vi "trace_viewer.vi"() -> ()   [LabVIEW 2012]
uses:
  testing/Trace controls.ctl
  testing/probe_point.ctl
  testing/flag_selector.ctl
  testing/status_flag.ctl
  testing/pose_selector.ctl
  testing/pose_source.ctl
  testing/pose_relative_to.ctl
  ltrace_index.ctl
  bool_condition.ctl
  <vilib>/Platform/TimedLoop/XDataNode/timing_clust.ctl
  <vilib>/Platform/TimedLoop/XDataNode/nitl_modes.ctl
  <vilib>/Platform/TimedLoop/XDataNode/wakeup.ctl
  <vilib>/Platform/TimedLoop/XDataNode/XDataNode.xnode
  <vilib>/Platform/TimedLoop/XDataNode/XDNodeRunTimeDep.lvlib
panel:
  in  "Max len":dbl=120.0
  out "Cursor time":timestamp
  out "Trace display":T1(graph)
  out "Progress":u8(slide) scale=0.0..100.0
  in  "Save trace":bool
  in  "Output path":path
  in  "Show":bool[](array[boolean])=[FALSE, FALSE, TRUE, TRUE, TRUE, FALSE, TRUE, TRUE, TRUE, TRUE, TRUE, FALSE, FALSE, FALSE, FALSE, FALSE, TRUE, TRUE]
  in  "Test":T2[](array[typedef])=[enum."*", enum."1", enum."*", enum."*", enum."*", enum."*", enum."*", enum."*", enum."*", enum."*", enum."*", enum."*", enum."*", enum."*", enum."*", enum."*", enum."*", enum."*"]
  out "Flag names":string[](array[string])
  in  "After":dbl
  in  "Before":dbl
  out "Sequence error":bool
  out "Out of order":i32
  out "Missing":i32
  out "Chunk binary data file":path caption="selected path"
  out "Chunks":cluster{T3[]}[](array[cluster]) {"?"."Timestamp" format="%<%.3X>T"}
  in  "Chunk browser":i32(listbox)
  out "File exists":bool
  in  "Input file":path
  in  "stop":bool
  in  "Reference hold":bool
  in  "Pose selectors":T4[](array[typedef])
  in  "Flag selectors":T7[](array[typedef])=[{"Flag"=enum."Cancellation", "Select"=TRUE}, {"Flag"=enum."Goal filter", "Select"=TRUE}, {"Flag"=enum."Valid position", "Select"=TRUE}, {"Flag"=enum."Velocity limiting", "Select"=TRUE}]
  in  "Decimate":i32=1 min=1 max=999 step=1
  out "2D position":cluster{"X":sgl[], "Y":sgl[]}[](graph)
  in  "Trace controls":T9[](array[typedef])=[{"+ stim"=FALSE, "Relative"=FALSE, "Scale"=enum."1X", "Probe point"=enum."Null pos (tip)", "XYZ selector"={"Boolean"=FALSE, "Boolean 2"=FALSE, "Boolean 3"=TRUE}, "To tip"=TRUE}, {"+ stim"=FALSE, "Relative"=FALSE, "Scale"=enum."1X", "Probe point"=enum."Goal (tip)", "XYZ selector"={"Boolean"=FALSE, "Boolean 2"=FALSE, "Boolean 3"=TRUE}, "To tip"=TRUE}, {"+ stim"=FALSE, "Relative"=FALSE, "Scale"=enum."1X", "Probe point"=enum."Position (tip)", "XYZ selector"={"Boolean"=FALSE, "Boolean 2"=FALSE, "Boolean 3"=TRUE}, "To tip"=TRUE}, {"+ stim"=FALSE, "Relative"=FALSE, "Scale"=enum."1X", "Probe point"=enum."Position (tip)", "XYZ selector"={"Boolean"=FALSE, "Boolean 2"=FALSE, "Boolean 3"=FALSE}, "To tip"=FALSE}]
  # "Trace Display"
  # "Chunk filtering"
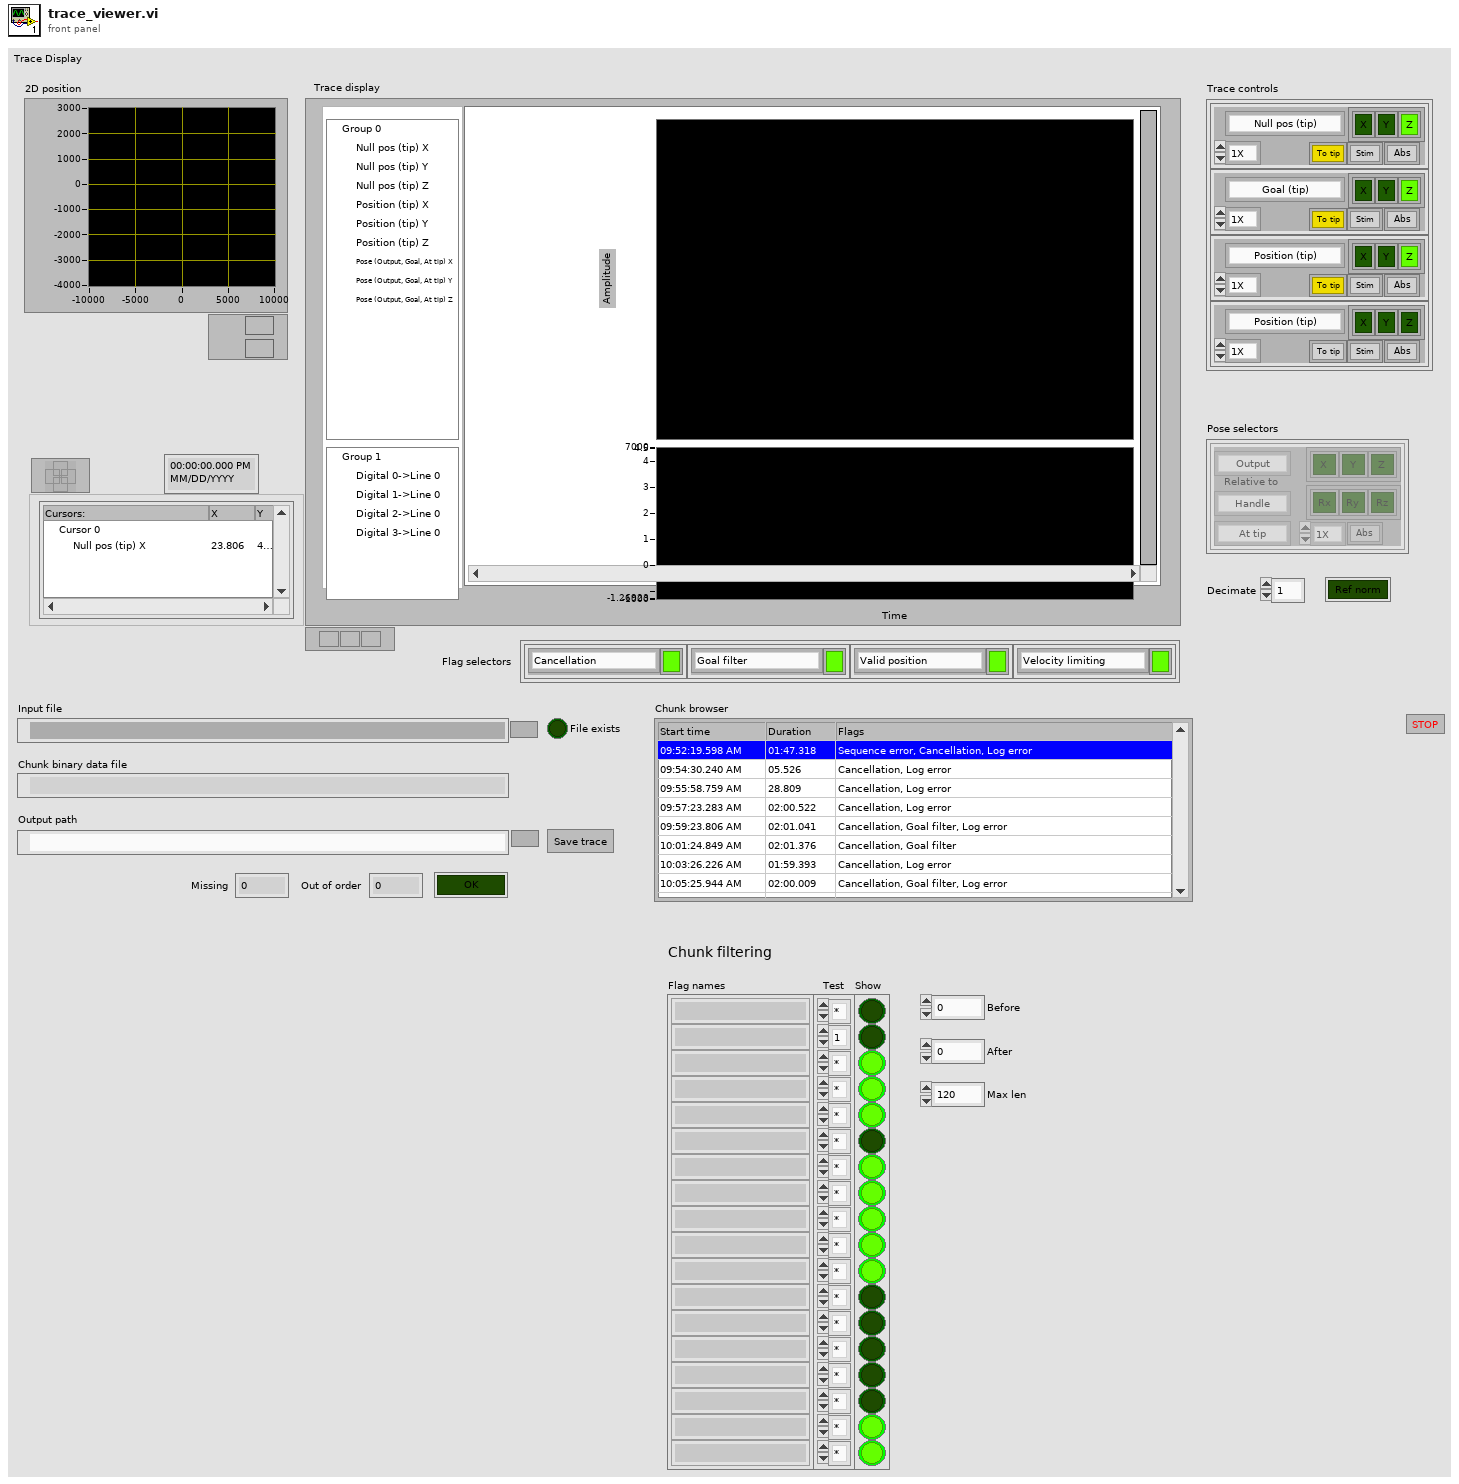
[diagram p1: front panel]
types:
  T1 = cluster{"Waveforms out":waveform(sgl)[], "Digital waveforms":digitalwaveform[]}
  T2 = typedef "bool_condition.ctl" = enum16{"0", "1", "*"}
  T3 = typedef "ltrace_index.ctl" = cluster{"Timestamp":timestamp, "Offset":i64, "Sequence":u32, "Flags":u32}
  T4 = typedef "pose_selector.ctl" = cluster{"Scale":enum16{"1X", "10X", "100X", "1KX", "10KX"}, "Source":T5, "XYZ selector":cluster{"Boolean":bool, "Boolean 2":bool, "Boolean 3":bool}, "RPY selector":cluster{"Boolean":bool, "Boolean 2":bool, "Boolean 3":bool}, "Relative to":T6, "Relative":bool, "Translate":enum16{"At tip", "At RCM", "At KC", "At origin"}}
  T5 = typedef "pose_source.ctl" = enum16{"Output", "Handle", "Handle KF", "Goal", "Absolute"}
  T6 = typedef "pose_relative_to.ctl" = enum16{"Output", "Handle", "Handle KF", "Goal", "Absolute", "Trace start"}
  T7 = typedef "flag_selector.ctl" = cluster{"Flag":T8, "Select":bool}
  T8 = typedef "status_flag.ctl" = enum16{"Cancellation", "Goal filter", "Valid position", "Goal saturation tip", "Goal saturation RCM", "Goal circle saturation", "Position saturation", "Output saturation", "Acceleration limiting", "Finished late", "Stimulus increasing", "Integral error saturation", "Velocity limiting", "Log warning", "Log error", "Link KF degraded"}
  T9 = typedef "Trace controls.ctl" = cluster{"+ stim":bool, "Relative":bool, "Scale":enum16{"1X", "10X", "100X", "1KX", "10KX"}, "Probe point":T10, "XYZ selector":cluster{"Boolean":bool, "Boolean 2":bool, "Boolean 3":bool}, "To tip":bool}
  T10 = typedef "probe_point.ctl" = enum16{"Position (tip)", "Position (RCM)", "Null pos (tip)", "Null pos (RCM)", "V limiter (tip)", "V Limiter (RCM)", "Goal (tip)", "Goal (RCM)", "Link pos 0", "Link pos 1", "KF link pos 0", "KF link pos 1", "Link rate 0", "Link rate 1", "Link residue 0", "Link residue 1", "Link goal 0", "Link goal 1", "Rate limit 0", "Rate limit 1", "Link error 0", "Link error 1", "Controller 0", "Controller 1", "Output 0", "Output 1", "Drive 0", "Drive 1", "Stimulus 0", "Stimulus 1", "Trace data 0", "Trace data 1", "Analog data 0", "Analog data 1", "Status flags", "Light 0", "Light 1", "Light 2", "Light 3", "Light 4", "Light 5", "Goal origin", "Goal rotation 0", "Goal rotation 1", "Goal rotation 2", "Output origin", "Output rotation 0", "Output rotation 1", "Output rotation 2", "Handle origin", "Handle rotation 0", "Handle rotation 1", "Handle rotation 2", "Handle position", "Handle velocity", "Handle acceleration", "Handle angles", "Handle angle rates", "Handle pos residue", "Handle angle residue", "Trace length"}
  T11 = typedef "XDNodeRunTimeDep.lvlib/timing_clust.ctl" = cluster{"Expected End [f-1]":u64, "Actual End [f-1]":u64, "Finished Late? [f-1]":bool, "Expected End [i-1]":u64, "Actual End [i-1]":u64, "Finished Late? [i-1]":bool, "Expected Start [i]":u64, "Actual Start [i]":u64, "Expected Start [f]":u64, "Actual Start [f]":u64, "Source Name":string, "Structure Name":string, "Period":i64, "Deadline":i64, "Offset":i64, "Start":i64, "Priority":i32, "Timeout":i32, "Mode":T12, "Wakeup Reason":T13, "Error":errorcluster, "Source Type":string, "Secondary Source Type":string, "Global End Time":u64, "Global Start Time":u64, "Frame Duration":u64, "Iteration Duration":u64, "Assigned CPU":i32, "I/O Scan Engine Mode":u32}
  T12 = typedef "XDNodeRunTimeDep.lvlib/nitl_modes.ctl" = enum32{"No Change", "Process missed periods, maintain original phase", "Discard missed periods, maintain original phase", "Process missed periods, ignore original phase", "Discard missed periods, ignore original phase"}
  T13 = typedef "XDNodeRunTimeDep.lvlib/wakeup.ctl" = enum32{"Normal", "Aborted", "Asynchronous wakeup", "Timing source error", "Timed loop error", "Timeout"}
  T14 = enum8{"Enabled", "Disabled", "Disabled and Grayed Out"}
  T15 = cluster{"Show":bool[], "Test":T2[], "After":dbl, "Before":dbl, "Max len":dbl}
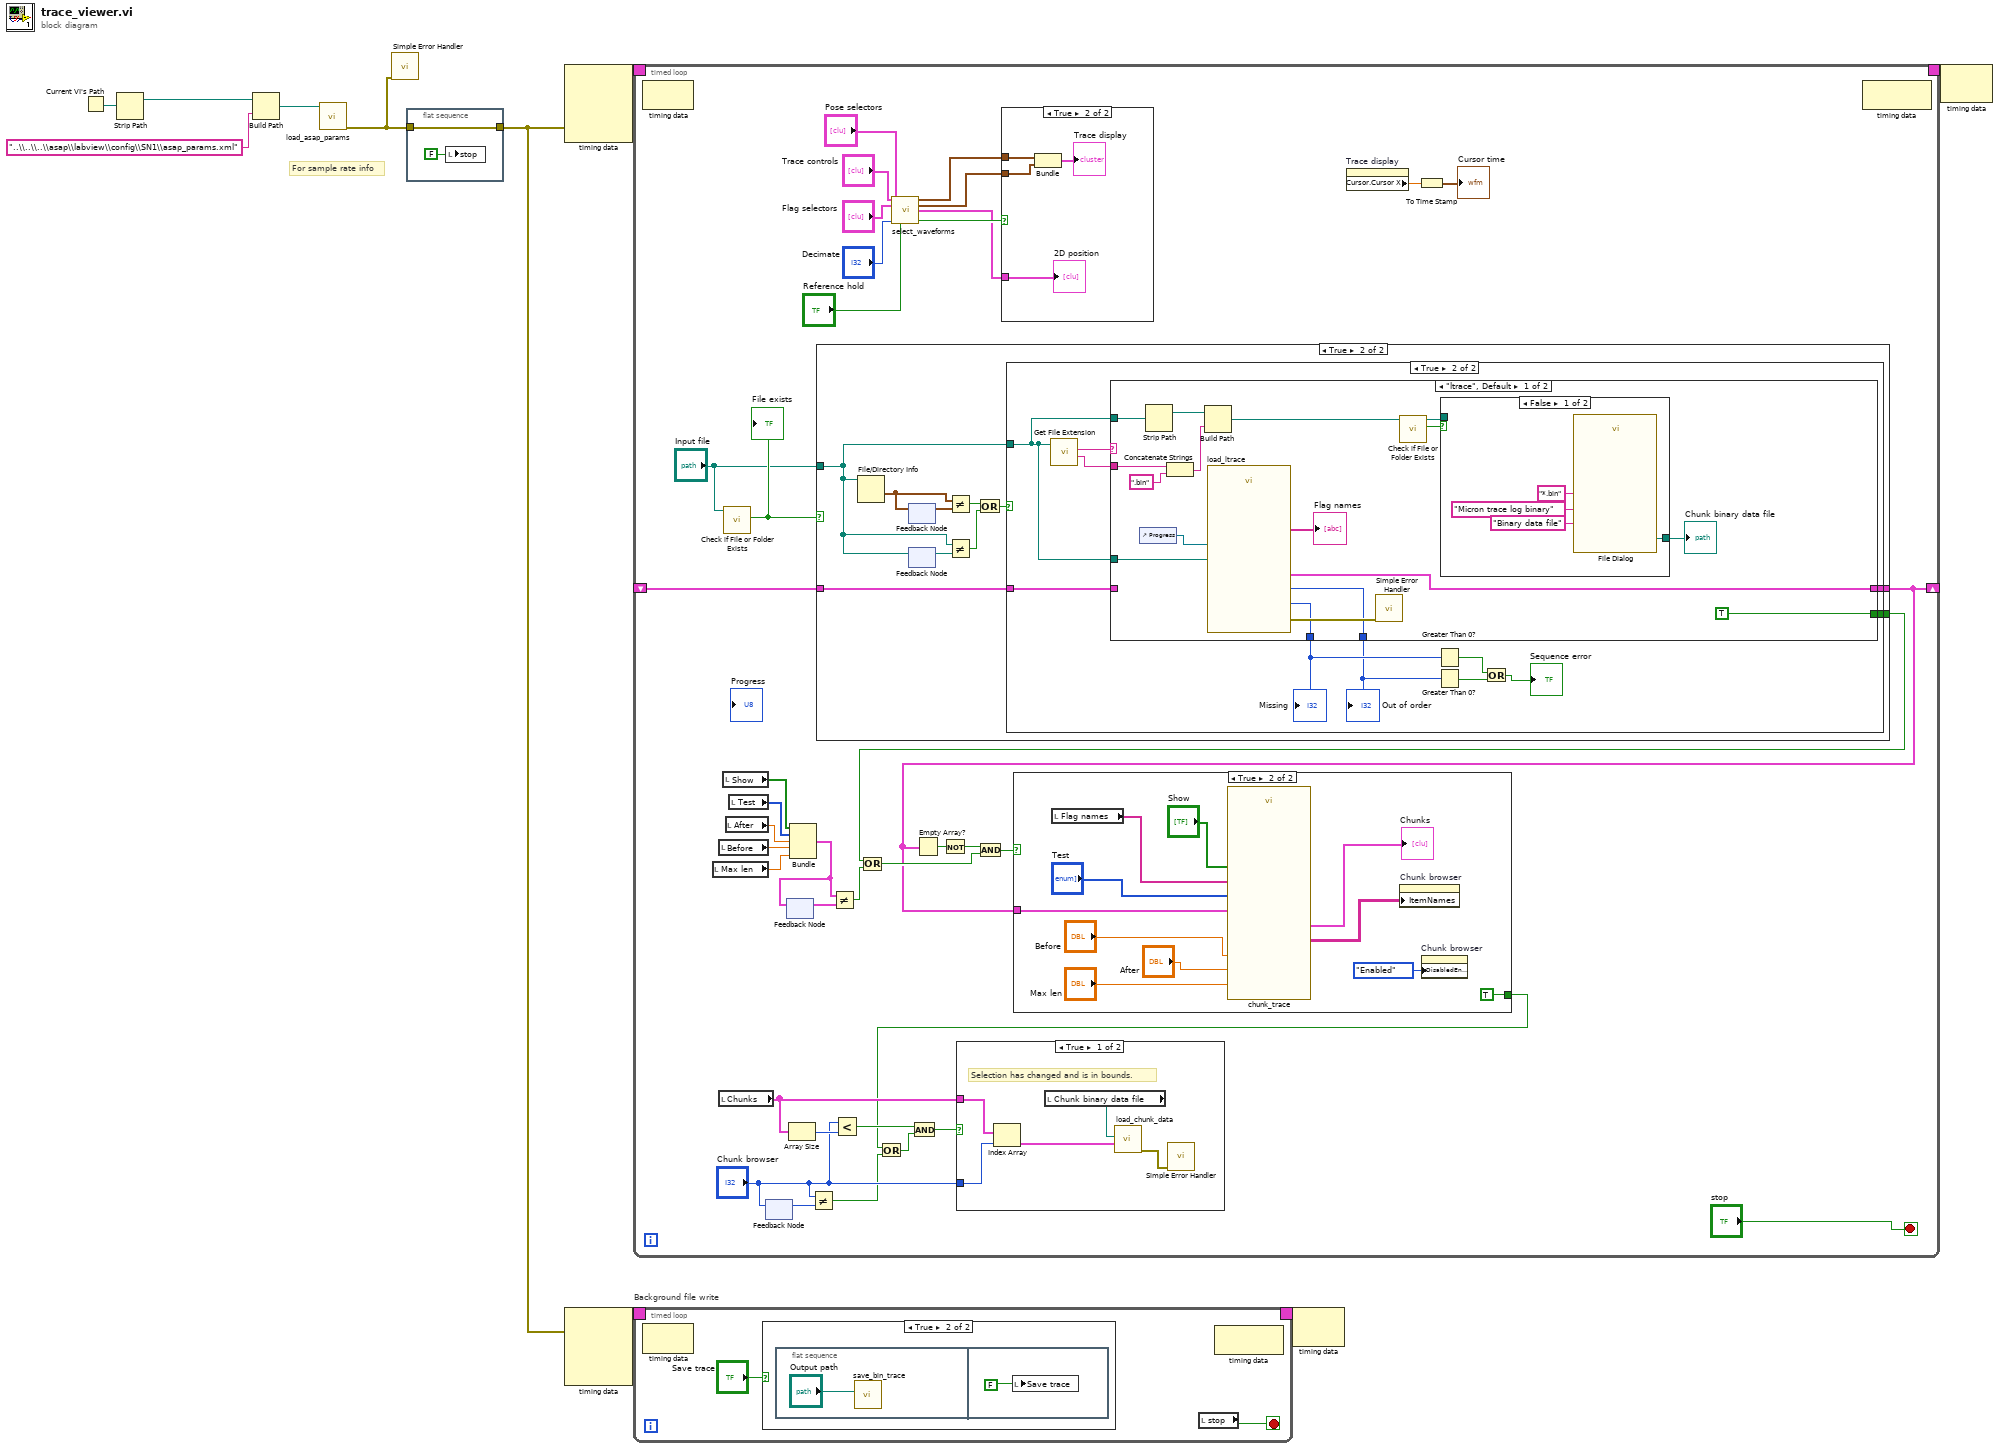
[diagram p0: block diagram]
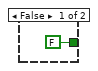
[diagram p3: hidden frame]
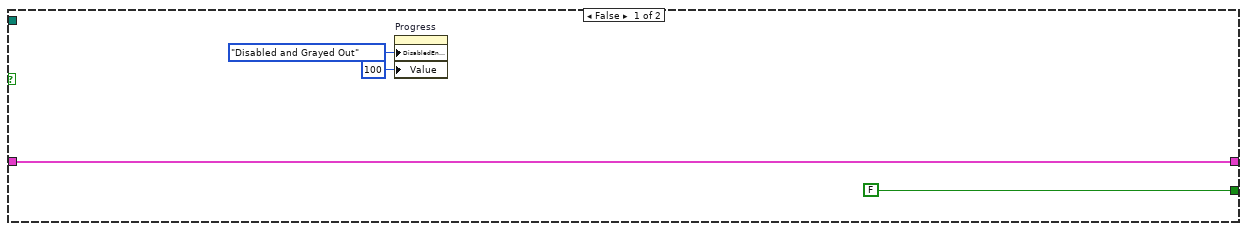
[diagram p5: hidden frame]
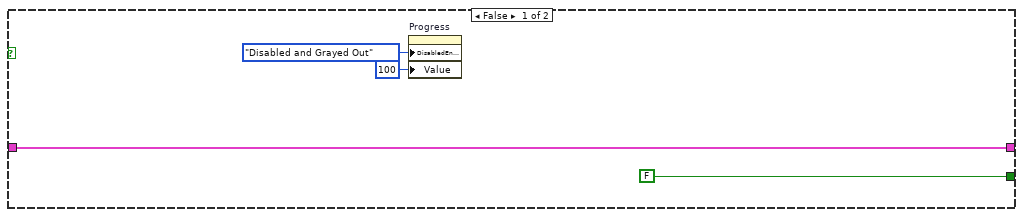
[diagram p6: hidden frame]
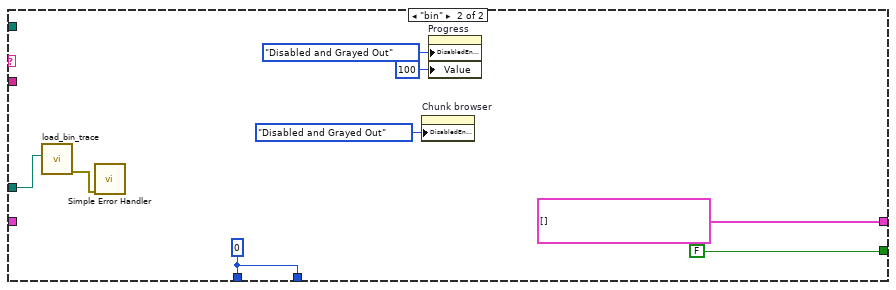
[diagram p8: hidden frame]
diagram:
  # "For sample rate info"
  n1 = Current VI's Path() -> (path=w5:path)
  n2 = Strip Path(path=w5) -> (stripped path=w4:path)  [unwired: 1 out]
  n3 = Build Path(base path=w4, name or relative path="..\\..\\..\\asap\\labview\\config\\SN1\\asap_params.xml") -> (appended path=w2:path)
  n4 = call "load_asap_params.vi"("ASAP params file"=w2) -> ("error out"=w1:errorcluster)  [unwired: 10 in]
  n5 = call <vilib>:"Simple Error Handler.vi"("error in (no error)"=w1) -> ()  [unwired: 4 in, 5 out]
  n6 = flat-sequence {
    tunnel: [w12] -> w6
    tunnel: w1 -> [w12]
    frame #0 {
      n7 = local write "stop"(FALSE ("stop")) -> ()
    }
  }
  n8 = node-c288(w6) -> (w10:T11)  [unwired: 3 in]
  n9 = node-c288(w6) -> (w8:T11)  [unwired: 3 out]
  n10 = timed-loop {
    timing: w10 -> [_]
    timing-out: [_] -> w9
    shift-right: [w33] -> _
    shift-left: _ -> [w39]
    stop <- "stop" stop-if-true
    n11 = node-c288() -> ()  [unwired: 1 in, 1 out]
    n12 = local read "Max len"() -> (w13:dbl)
    n13 = local read "Before"() -> (w28:dbl)
    n14 = local read "Chunks"() -> (w24:cluster{T3[]}[])
    n15 = local read "Show"() -> (w26:bool[])
    n16 = call <vilib>:"Check if File or Folder Exists.vi"("path"="Input file") -> ("file or folder exists?"=w41:bool)  [unwired: 8 in, 2 out]
    "File exists" <- w41
    n17 = local read "After"() -> (w29:dbl)
    n18 = local read "Test"() -> (w30:T2[])
    n19 = feedback #1() -> (w25:i32)  [unwired: 1 in]
    n20 = feedback-in #1("Chunk browser") -> ()
    n21 = feedback #2() -> (w38:T15)  [unwired: 1 in]
    n22 = Array Size(array=w24) -> (size(s)=w23:i32)
    n23 = Bundle("Show"=w26, "Test"=w30, "After"=w29, "Before"=w28, "Max len"=w13) -> (w27:T15)  [unwired: 1 in]
    n24 = feedback-in #2(w27) -> ()
    n25 = Not Equal?(x="Chunk browser", y=w25) -> (x != y?=w18:bool)
    n26 = case shown="True" w41 {
      tunnel: "Input file" -> [_ w78]
      tunnel: w39 -> [w71 w74]
      tunnel: [w71 w73] -> w33
      tunnel: [FALSE ("x .or. y?") w72] -> w34
      frame False {
        n27 = property on="Progress" class="Slide (strict)"("DisabledEnum"=T14."Disabled and Grayed Out" ("Disabled"), "Value"=u8 100 ("Progress")) -> ()  [unwired: 2 in, 2 out]
      }
      frame True {
        n28 = File/Directory Info(path=w78) -> (last mod=w79:timestamp)  [unwired: 1 in, 6 out]
        n29 = feedback #3() -> (w80:timestamp)  [unwired: 1 in]
        n30 = feedback-in #3(w79) -> ()
        n31 = feedback #4() -> (w81:path)  [unwired: 1 in]
        n32 = feedback-in #4(w78) -> ()
        n33 = Not Equal?(x=w79, y=w80) -> (x != y?=w77:bool)
        n34 = Not Equal?(x=w78, y=w81) -> (x != y?=w76:bool)
        n35 = Or(x=w77, y=w76) -> (x .or. y?=w75:bool)
        n36 = case shown="True" w75 {
          tunnel: w78 -> [_ w86]
          tunnel: w74 -> [w85 w89]
          tunnel: [w85 w88] -> w73
          tunnel: [FALSE ("x .or. y?") w87] -> w72
          frame False {
            n37 = property on="Progress" class="Slide (strict)"("DisabledEnum"=T14."Disabled and Grayed Out" ("Disabled"), "Value"=u8 100 ("Progress")) -> ()  [unwired: 2 in, 2 out]
          }
          frame True {
            n38 = call <vilib>:"Get File Extension.vi"("file"=w86) -> ("filename without extension"=w95:string, "lowercase file extension"=w96:string)  [unwired: 7 in, 2 out]
            n39 = case shown="\"ltrace\", Default" w96 {
              tunnel: w86 -> [w113 w126]
              tunnel: w95 -> [w111 _]
              tunnel: [w106 w124] -> w94
              tunnel: [w105 w124] -> w93
              tunnel: w89 -> [_ _]
              tunnel: [w104 T3[] [] ("File index")] -> w88
              tunnel: [TRUE ("x .or. y?") FALSE ("x .or. y?")] -> w87
              tunnel: w86 -> [w102 _]
              frame "ltrace", Default {
                n40 = control-ref of="Progress"() -> (w98:refnum<vi>)
                n41 = Strip Path(path=w102) -> (stripped path=w101:path)  [unwired: 1 out]
                n42 = Concatenate Strings(w111, ".bin" ("string")) -> (w100:string)
                n43 = Build Path(base path=w101, name or relative path=w100) -> (appended path=w99:path)
                n44 = call "load_ltrace.vi"("Progress"=w98, "File path"=w113) -> ("error out"=w107:errorcluster, "File index"=w104:T3[], "Out of order"=w105:i32, "Flag names"=→"Flag names":string[], "Missing"=w106:i32)  [unwired: 5 in]
                n45 = call <vilib>:"Simple Error Handler.vi"("error in (no error)"=w107) -> ()  [unwired: 4 in, 5 out]
                n46 = call <vilib>:"Check if File or Folder Exists.vi"("path"=w99) -> ("file or folder exists?"=w109:bool, "dup path"=w108:path)  [unwired: 8 in, 1 out]
                n47 = case shown="False" w109 {
                  tunnel: [w114 w118] -> w110
                  tunnel: w108 -> [_ w118]
                  frame False {
                    n48 = call "File Dialog"("prompt"="Binary data file", "pattern (all files)"="*.bin", "pattern label"="Micron trace log binary") -> ("selected path"=w114:path)  [unwired: 9 in, 3 out]
                  }
                  frame True {
                  }
                }
                "Chunk binary data file" <- w110
              }
              frame "bin" {
                w124 = 0 ("Missing")
                n49 = call "load_bin_trace.vi"("File path"=w126) -> ("error out"=w125:errorcluster)  [unwired: 9 in, 1 out]
                n50 = call <vilib>:"Simple Error Handler.vi"("error in (no error)"=w125) -> ()  [unwired: 4 in, 5 out]
                n51 = property on="Chunk browser" class="MCListbox (strict)"("DisabledEnum"=T14."Disabled and Grayed Out" ("Disabled")) -> ()  [unwired: 2 in, 2 out]
                n52 = property on="Progress" class="Slide (strict)"("DisabledEnum"=T14."Disabled and Grayed Out" ("Disabled"), "Value"=u8 100 ("Progress")) -> ()  [unwired: 2 in, 2 out]
              }
            }
            "Missing" <- w94
            "Out of order" <- w93
            n53 = Greater Than 0?(x=w94) -> (x > 0?=w92:bool)
            n54 = Greater Than 0?(x=w93) -> (x > 0?=w91:bool)
            n55 = Or(x=w92, y=w91) -> (x .or. y?=→"Sequence error":bool)
          }
        }
      }
    }
    n56 = Not Equal?(x=w27, y=w38) -> (x != y?=w36:bool)
    n57 = Less?(x="Chunk browser", y=w23) -> (x < y?=w21:bool)
    n58 = Or(x=w34, y=w36) -> (x .or. y?=w35:bool)
    n59 = call "select_waveforms.vi"("Trace controls"="Trace controls", "Flag selectors"="Flag selectors", "Pose selectors"="Pose selectors", "Decimate"="Decimate", "Reference hold"="Reference hold") -> ("Waveforms out"=w14:waveform(sgl)[], "Digital waveforms"=w47:digitalwaveform[], "XY views"=w48:cluster{"X":sgl[], "Y":sgl[]}[], "New data"=w49:bool)  [unwired: 7 in]
    n60 = Empty Array?(array=w33) -> (empty?=w32:bool)
    n61 = Not(x=w32) -> (.not. x?=w31:bool)
    n62 = And(x=w31, y=w35) -> (x .and. y?=w37:bool)
    n63 = case shown="True" w49 {
      tunnel: w14 -> [_ w129]
      tunnel: w48 -> [_ w130]
      tunnel: w47 -> [_ w128]
      frame False {
      }
      frame True {
        n64 = Bundle("Waveforms out"=w129, "Digital waveforms"=w128) -> (→"Trace display":T1)  [unwired: 1 in]
        "2D position" <- w130
      }
    }
    n65 = case shown="True" w37 {
      tunnel: w33 -> [_ w60]
      tunnel: [FALSE ("x != y?") TRUE ("x != y?")] -> w17
      frame False {
      }
      frame True {
        n66 = local read "Flag names"() -> (w54:string[])
        n67 = call "chunk_trace.vi"("After"="After", "Note"="Show", "Before"="Before", "Flag names"=w54, "Max len"="Max len", "Condition"="Test", "Index array"=w60) -> ("Descriptions"=w61:string[][], "Chunks"=→"Chunks":cluster{T3[]}[])  [unwired: 3 in]
        n68 = property on="Chunk browser" class="MCListbox (strict)"("ItemNames"=w61) -> ()  [unwired: 2 in, 2 out]
        n69 = property on="Chunk browser" class="MCListbox (strict)"("DisabledEnum"=T14."Enabled" ("Disabled")) -> ()  [unwired: 2 in, 2 out]
      }
    }
    n70 = Or(x=w17, y=w18) -> (x .or. y?=w19:bool)
    n71 = And(x=w21, y=w19) -> (x .and. y?=w20:bool)
    n72 = case shown="True" w20 {
      tunnel: "Chunk browser" -> [w67 _]
      tunnel: w24 -> [w63 _]
      frame True {
        # "Selection has changed and is in bounds."
        n73 = Index Array(array=w63, index=w67) -> (element=w66:cluster{T3[]})
        n74 = local read "Chunk binary data file"() -> (w65:path)
        n75 = call "load_chunk_data.vi"("Chunk"=w66, "File path"=w65) -> ("error out"=w64:errorcluster)  [unwired: 8 in, 1 out]
        n76 = call <vilib>:"Simple Error Handler.vi"("error in (no error)"=w64) -> ()  [unwired: 4 in, 5 out]
      }
      frame False {
        # "No change in selection or out of bounds"
      }
    }
    n77 = property on="Trace display" class="MixedGraph (strict)"() -> ("Cursor.Cursor X"=w16:dbl)  [unwired: 2 in, 2 out]
    n78 = To Time Stamp(1:w16) -> (0:→"Cursor time":timestamp)
    n79 = node-c288() -> ()  [unwired: 1 in, 1 out]
  }
  n80 = timed-loop "Background file write" {
    timing: w8 -> [_]
    timing-out: [_] -> w7
    stop <- w133 stop-if-true
    n81 = node-c288() -> ()  [unwired: 2 out]
    n82 = case shown="True" "Save trace" {
      frame False {
      }
      frame True {
        n83 = flat-sequence {
          frame #0 {
            n84 = call "save_bin_trace.vi"("File path"="Output path") -> ()  [unwired: 1 in, 10 out]
          }
          frame #1 {
            n85 = local write "Save trace"(FALSE ("Save trace")) -> ()
          }
        }
      }
    }
    n86 = local read "stop"() -> (w133:bool)
    n87 = node-c288() -> ()  [unwired: 2 out]
  }
  n88 = node-c288(w7) -> ()  [unwired: 1 out]
  n89 = node-c288(w9) -> ()  [unwired: 1 out]
